vi "Insert Error.vi"(8 "error in":errorcluster, 11 "Error Code":i32) -> (0 "error out":errorcluster)   [LabVIEW 2017, in "TSC Error.lvlib"]
doc: "This VI will add an error to the error wire. This is an easy way to set a custom error in the application.\n\nInputs:\n-Error Code [I32] - the error code to insert\n-error in\n\nOutputs:\n-error out\n\n______________________________________\n<b>Code Developed By:</b>\nDaniel Coons\nTechnology Service Corporation\n1983 S Liberty Drive\nBloomington, IN 47403\nPhone: 812 558-7100\ndaniel.coons@tsc.com\nwww.tsc.com\n\n<b>Date Created:</b> 11 AUG 2014\n<b>Date Updated:</b>"
uses:
  TSC Error.lvlib
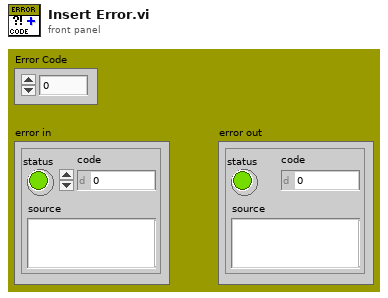
[diagram p1: front panel]
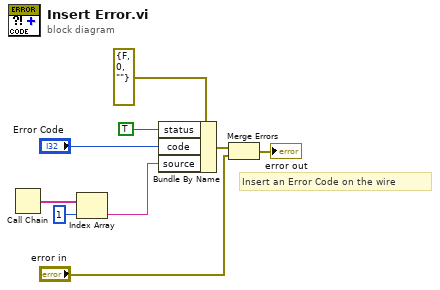
[diagram p0: block diagram]
diagram:
  # "Insert an Error Code on the wire"
  n1 = Call Chain() -> (call chain=w3:string[])
  n2 = Index Array "Index Array"(array=w3, index=1) -> (element=w1:string)
  n3 = Bundle By Name(cluster=errorcluster {"status"=FALSE, "code"=0, "source"=""} ("t"), "status"=TRUE, "code"="Error Code", "source"=w1) -> (w5:errorcluster)
  n4 = Merge Errors(w5, "error in") -> (→"error out":errorcluster)
